vi "2D__Scaner+FM_v.9.6-ESP32.vi"() -> ()   [LabVIEW 2018]
uses:
  <vilib>/Analysis/Matrix/Datatypes/RealMatrix.ctl
  <vilib>/Platform/TimedLoop/XDataNode/timing_clust.ctl
  <vilib>/Platform/TimedLoop/XDataNode/nitl_modes.ctl
  <vilib>/Platform/TimedLoop/XDataNode/wakeup.ctl
  GlobalStop.vi
  <vilib>/Platform/TimedLoop/XDataNode/XDataNode.xnode
  <vilib>/Platform/TimedLoop/XDataNode/XDNodeRunTimeDep.lvlib
  <vilib>/Analysis/Matrix/NI_Matrix.lvlib
panel:
  out "Hour":i32 caption="Оставшееся время"
  out "Min":i32 caption="Оставшееся время"
  in  "Att":dbl(ring)=1.0 caption="Аттенюатор" items=["None"=1.0, "1%"=100.0, "3%"=34.0, "10%"=13.5, "30%"=4.6, "1+3%"=3400.0, "1+10%"=1350.0, "1+30%"=460.0, "3+10%"=459.0, "3+30%"=156.4, "10+30%"=62.1, "1+3+10%"=45900.0, "1+3+30%"=15640.0, "1+10+30%"=6210.0, "3+10+30%"=2111.4, "All"=211140.0]
  in  "Reboot ESP":bool
  out "Dir_x":bool
  out "Y_iter":i32
  in  "X_iter":i32
  in  "calc fi":bool=TRUE caption="Пересчет\nX в fi"
  out "pos_xy":cluster{"pos_x":dbl, "pos_y":dbl} caption="Позиция 2D, мм"
  in  "Mode initial 2D":enum32{"2D", "X"}(radio)=enum."X"
  out "pos_sample":dbl caption="Позиция FM с образцом"
  out "pos_no_sample":dbl caption="Позиция FM без образца"
  in  "Check pos":bool
  out "Sec":i32 caption="Оставшееся время"
  in  "Режим\nсканирования":enum32{"Ampl", "Phase"}(radio)
  out "st_joy":bool
  in  "Джостик":bool
  in  "Left":bool
  in  "Up":bool
  in  "Down":bool
  in  "Right":bool
  in  "Шаг, мкм":dbl=10000.0
  in  "Find pp":bool
  in  "Толщина образца":dbl min=0.0
  out "P_ref":dbl caption="Опорный сигнал \nс детектора"
  out "error sign.detect":errorcluster
  out "error esp-32":errorcluster
  out "COM-port":refnum<visa-resource-name>
  in  "COM-port ESP-32":refnum<visa-resource-name>="COM3"
  out "error out":errorcluster
  in  "error in (no error)":errorcluster
  in  "read signal?":bool
  in  "К позиции FM":i32=1000
  in  "Rotate FM":bool
  out "pos_z":dbl caption="Позиция FM"
  in  "Initial FM":bool
  out "График интенсивности":dbl[][](graph)
  in  "стоп":bool
  out "Завершено, %":dbl(slide) scale=0.0..100.0
  in  "Шаг по X":u32(knob)=1000 max=20000 scale=1.0..1000.0 scale format="%.0p"
  in  "начало Y, мм":dbl
  in  "начало X, мм":dbl
  in  "конец Y, мм":dbl=1.0
  in  "конец X, мм":dbl=1.0
  out "Результат сканирования":T1
  in  "Комментарий к файлу":string=" "
  in  "отмена":bool
  in  "сохр":bool
  in  "Имя файла с результатами":path=path "results.lvm" caption="Filename"
  in  "start scaning":bool
  in  "Шаг по Y":u32(knob)=1000 max=10000 scale=10.0..1000.0 scale format="%3.0p"
  out "Диалоговое окно":string
  in  "Initial 2D":bool
  in  "Частота излучения":dbl min=0.001
  # "Оставшееся время"
  # "м"
  # "с"
  # "ч"
  # "мм"
  # "Параметры сканирования"
  # "Начальная \nпозиция"
  # "ГГц"
  # "Область\nсканирования"
  # "мкм"
  # "Конечная\nпозиция"
  # "мм"
  # "мм"
  # "мм"
  # "мкм"
  # "мкм"
  # "мкм"
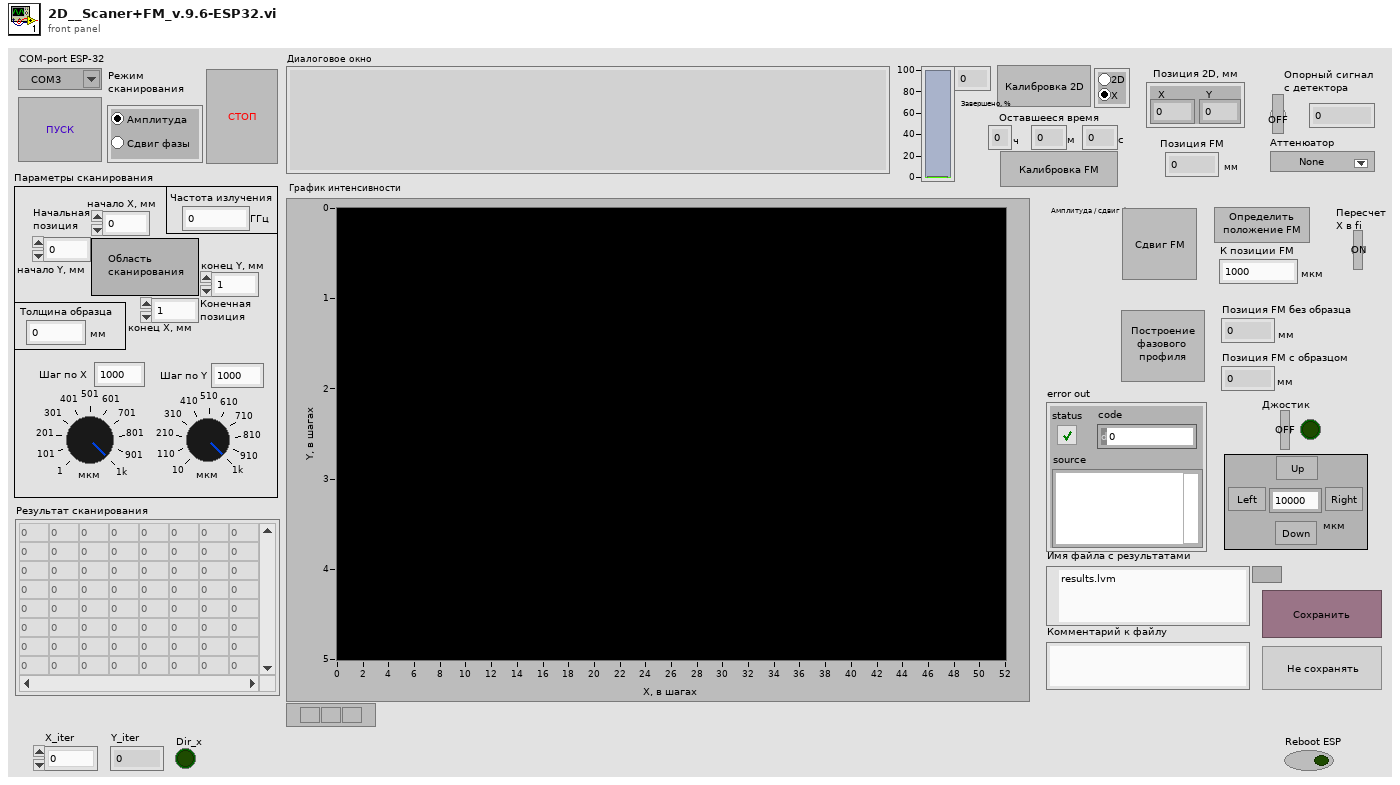
[diagram p1: front panel]
types:
  T1 = typedef "NI_Matrix.lvlib/RealMatrix.ctl" = dbl[][]
  T2 = typedef "XDNodeRunTimeDep.lvlib/timing_clust.ctl" = cluster{"Expected End [f-1]":u64, "Actual End [f-1]":u64, "Finished Late? [f-1]":bool, "Expected End [i-1]":u64, "Actual End [i-1]":u64, "Finished Late? [i-1]":bool, "Expected Start [i]":u64, "Actual Start [i]":u64, "Expected Start [f]":u64, "Actual Start [f]":u64, "Source Name":string, "Structure Name":string, "Period":i64, "Deadline":i64, "Offset":i64, "Start":i64, "Priority":i32, "Timeout":i32, "Mode":T3, "Wakeup Reason":T4, "Error":errorcluster, "Source Type":string, "Secondary Source Type":string, "Global End Time":u64, "Global Start Time":u64, "Frame Duration":u64, "Iteration Duration":u64, "Assigned CPU":i32, "I/O Scan Engine Mode":u32}
  T3 = typedef "XDNodeRunTimeDep.lvlib/nitl_modes.ctl" = enum32{"No Change", "Process missed periods, maintain original phase", "Discard missed periods, maintain original phase", "Process missed periods, ignore original phase", "Discard missed periods, ignore original phase"}
  T4 = typedef "XDNodeRunTimeDep.lvlib/wakeup.ctl" = enum32{"Normal", "Aborted", "Asynchronous wakeup", "Timing source error", "Timed loop error", "Timeout"}
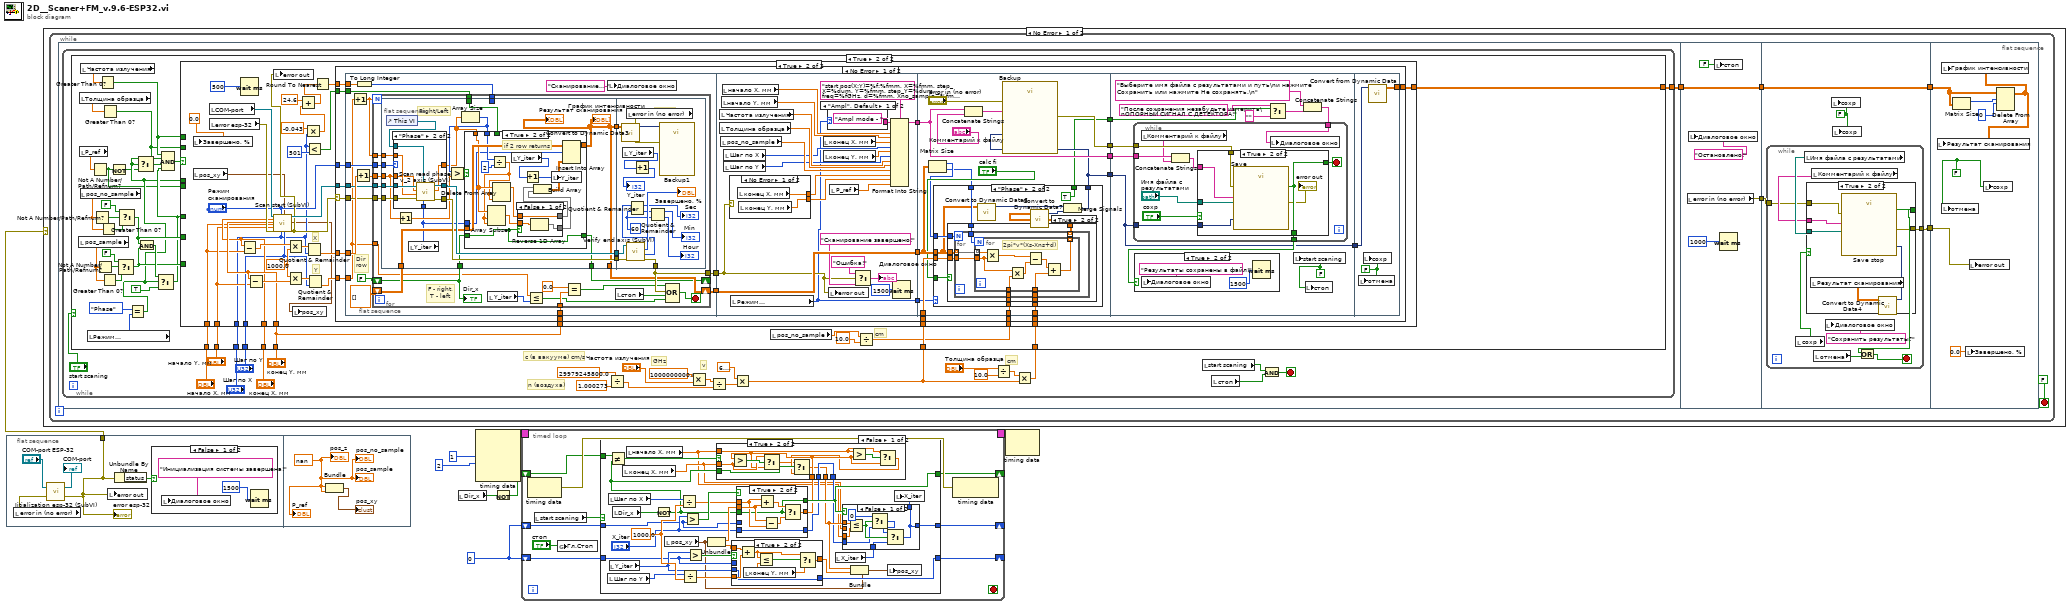
[diagram p0: block diagram]
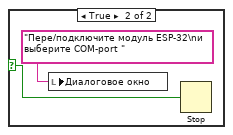
[diagram p2: hidden frame]
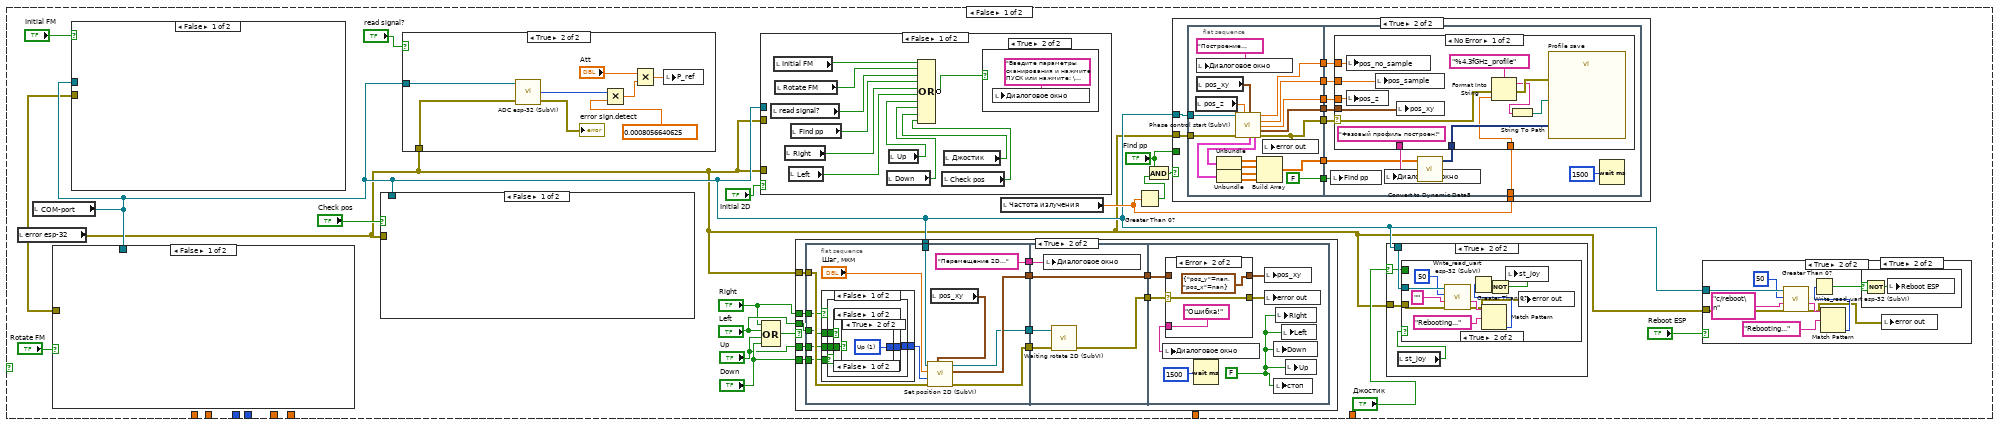
[diagram p3: hidden frame]
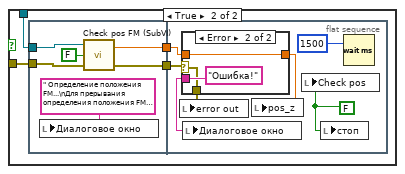
[diagram p6: hidden frame]
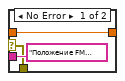
[diagram p7: hidden frame]
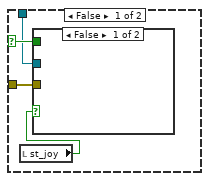
[diagram p8: hidden frame]
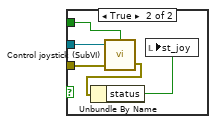
[diagram p9: hidden frame]
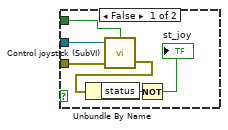
[diagram p10: hidden frame]
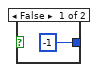
[diagram p12: hidden frame]
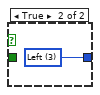
[diagram p13: hidden frame]
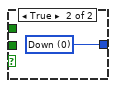
[diagram p14: hidden frame]
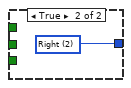
[diagram p15: hidden frame]
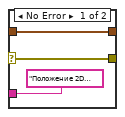
[diagram p16: hidden frame]
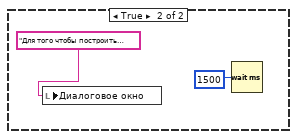
[diagram p18: hidden frame]
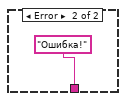
[diagram p19: hidden frame]
diagram:
  w3 = 0 ("Y_iter")
  n1 = flat-sequence {
    tunnel: [w9] -> w6
    frame #0 {
      n2 = local read "error in (no error)"() -> (w11:errorcluster)
      n3 = call "Iitialization esp-32 (SubVI).vi"("error in (no error)"=w11, "COM-port"="COM-port ESP-32") -> ("error out"=w9:errorcluster, "COM-port out"=→"COM-port":refnum<visa-resource-name>)
      "error esp-32" <- w9
      n4 = local write "error out"(w9) -> ()
      n5 = Unbundle By Name(w9) -> ("status"=w10:bool)
      n6 = case shown="False" w10 {
        selector: w10 -> [_ w16]
        frame False {
          n7 = local write "Диалоговое окно"("Инициализация системы завершена!" ("Диалоговое окно")) -> ()
          n8 = Wait (ms)(milliseconds to wait=u32 1500) -> ()  [unwired: 1 out]
        }
        frame True {
          n9 = local write "Диалоговое окно"("Пере/подключите модуль ESP-32\nи выберите COM-port " ("t")) -> ()
          n10 = Stop(stop? (T)=w16) -> ()
        }
      }
    }
    frame #1 {
      w19 = nan
      n11 = Bundle(w19, w19) -> (→"pos_xy":cluster{dbl, dbl})  [unwired: 1 in]
      "pos_z" <- w19
      "P_ref" <- w19
      "pos_no_sample" <- w19
      "pos_sample" <- w19
    }
  }
  n12 = case shown="No Error" w6 {
    frame No Error {
      n13 = while {
        stop <- FALSE stop-if-true
        n14 = flat-sequence {
          tunnel: [w26] -> w22
          tunnel: w22 -> [w723]
          tunnel: [w723] -> w21
          tunnel: [w719] -> w20
          tunnel: [w727] -> w25
          tunnel: w21 -> [w727]
          tunnel: w20 -> [w725]
          tunnel: [w724] -> w23
          tunnel: w25 -> [w750]
          tunnel: w23 -> [w747]
          frame #0 {
            n15 = while {
              tunnel: [w49] -> w26
              stop <- w38 stop-if-true
              # "cm"
              # "v"
              # "GHz"
              # "n (воздуха)"
              # "c (в вакууме) cm/s"
              n16 = Divide(x=29979245800.0, y=1.000273) -> (x/y=w43:dbl)
              n17 = Multiply(x=1000000000.0, y="Частота излучения") -> (x*y=w34:dbl)
              n18 = Divide(x=w34, y=w43) -> (x/y=w31:dbl)
              n19 = Multiply(x=6.283185307179586, y=w31) -> (x*y=w32:dbl)
              n20 = Divide(x="Толщина образца", y=10.0) -> (x/y=w29:dbl)
              n21 = Multiply(x=w29, y=w32) -> (x*y=w42:dbl)
              n22 = case shown="True" "start scaning" {
                tunnel: "конец Y, мм" -> [_ w341]
                tunnel: "конец X, мм" -> [_ w346]
                tunnel: "начало Y, мм" -> [_ w343]
                tunnel: "начало X, мм" -> [_ w342]
                tunnel: [_ w371] -> w49
                tunnel: w32 -> [_ w370]
                tunnel: w42 -> [_ w369]
                tunnel: "Шаг по X" -> [_ w344]
                tunnel: "Шаг по Y" -> [_ w345]
                frame False {
                  n23 = local read "error esp-32"() -> (w51:errorcluster)
                  n24 = local read "COM-port"() -> (w52:refnum<visa-resource-name>)
                  n25 = case shown="False" "Rotate FM" {
                    tunnel: w52 -> [_ w256]
                    tunnel: w51 -> [_ w252]
                    frame False {
                    }
                    frame True {
                      n26 = flat-sequence {
                        tunnel: w256 -> [w264]
                        tunnel: w252 -> [w258]
                        tunnel: [w262] -> w255
                        tunnel: [w261] -> w254
                        tunnel: [FALSE ("Rotate FM")] -> w253
                        tunnel: w255 -> [w267]
                        tunnel: w254 -> [w266]
                        tunnel: w253 -> [w265]
                        frame #0 {
                          n27 = local write "Диалоговое окно"("Перемещение FM...\nДля прерывания перемещения FM нажмите на Джостик!" ("Диалоговое окно")) -> ()
                          n28 = local read "pos_z"() -> (w259:dbl)
                          n29 = call "Set position FM (SubVI).vi"("VISA Refnum in"=w264, "Позиция, мкм"="К позиции FM", "error in"=w258, "pos_z"=w259) -> ("set_pos_z"=w262:dbl, "error out"=w261:errorcluster)  [unwired: 2 in]
                        }
                        frame #1 {
                          n30 = local write "Rotate FM"(w265) -> ()
                          n31 = case shown="No Error" w266 {
                            selector: w266 -> [w272 w275]
                            tunnel: ["Положение FM достигнуто!" ("Диалоговое окно") "Ошибка!" ("Диалоговое окно")] -> w270
                            tunnel: w267 -> [w273 _]
                            tunnel: [w273 nan ("set_pos_x")] -> w268
                            tunnel: [w272 w275] -> w269
                            frame No Error {
                            }
                            frame Error {
                            }
                          }
                          n32 = local write "Диалоговое окно"(w270) -> ()
                          n33 = local write "error out"(w269) -> ()
                          n34 = local write "стоп"(w265) -> ()
                          n35 = local write "pos_z"(w268) -> ()
                          n36 = Wait (ms)(milliseconds to wait=u32 1500) -> ()  [unwired: 1 out]
                        }
                      }
                    }
                  }
                  n37 = case shown="False" "Initial FM" {
                    tunnel: w51 -> [_ w282]
                    tunnel: w52 -> [_ w281]
                    frame False {
                    }
                    frame True {
                      n38 = flat-sequence {
                        tunnel: w282 -> [w287]
                        tunnel: w281 -> [w286]
                        tunnel: [w285] -> w280
                        tunnel: [FALSE ("Initial FM")] -> w279
                        tunnel: [u32 1500 ("milliseconds to wait")] -> w278
                        tunnel: w280 -> [w292]
                        tunnel: w279 -> [w289]
                        tunnel: w278 -> [w291]
                        frame #0 {
                          n39 = local write "Диалоговое окно"("Калибровка FM...\nДля прерывания калибровки FM нажмите на Джостик!" ("Диалоговое окно")) -> ()
                          n40 = call "Initial Z (SubVI).vi"("error in (no error)"=w287, "VISA Refnum in"=w286) -> ("error out"=w285:errorcluster)  [unwired: 1 in]
                        }
                        frame #1 {
                          n41 = Wait (ms)(milliseconds to wait=w291) -> ()  [unwired: 1 out]
                          n42 = case shown="No Error" w292 {
                            selector: w292 -> [w297 w300]
                            tunnel: [w297 w300] -> w294
                            tunnel: ["Калибровка завершена!" ("Диалоговое окно") "Ошибка!" ("Диалоговое окно")] -> w290
                            tunnel: [0.0 nan] -> w293
                            frame No Error {
                            }
                            frame Error {
                            }
                          }
                          n43 = local write "Initial FM"(w289) -> ()
                          n44 = local write "Диалоговое окно"(w290) -> ()
                          n45 = local write "pos_z"(w293) -> ()
                          n46 = local write "стоп"(w289) -> ()
                          n47 = local write "error out"(w294) -> ()
                        }
                      }
                    }
                  }
                  n48 = case shown="False" "Check pos" {
                    tunnel: w52 -> [_ w83]
                    tunnel: w51 -> [_ w82]
                    frame False {
                    }
                    frame True {
                      n49 = flat-sequence {
                        tunnel: w83 -> [w89]
                        tunnel: w82 -> [w88]
                        tunnel: [w87] -> w81
                        tunnel: [w86] -> w80
                        tunnel: w81 -> [w96]
                        tunnel: w80 -> [w95]
                        frame #0 {
                          n50 = local write "Диалоговое окно"(" Определение положения FM...\nДля прерывания определения положения FM нажмите на Джостик!" ("Диалоговое окно")) -> ()
                          n51 = call "Check pos FM (SubVI).vi"("error in"=w88, "verify?"=FALSE, "VISA Refnum in"=w89) -> ("error out"=w87:errorcluster, "position"=w86:dbl)
                        }
                        frame #1 {
                          w91 = FALSE
                          n52 = case shown="Error" w96 {
                            selector: w96 -> [w98 w101]
                            tunnel: ["Положение FM определено!" ("Диалоговое окно") "Ошибка!" ("Диалоговое окно")] -> w93
                            tunnel: [w97 w100] -> w94
                            tunnel: [w98 w101] -> w90
                            tunnel: w95 -> [w97 w100]
                            frame No Error {
                            }
                            frame Error {
                            }
                          }
                          n53 = local write "error out"(w90) -> ()
                          n54 = local write "Диалоговое окно"(w93) -> ()
                          n55 = local write "pos_z"(w94) -> ()
                          n56 = local write "Check pos"(w91) -> ()
                          n57 = local write "стоп"(w91) -> ()
                          n58 = Wait (ms)(milliseconds to wait=u32 1500) -> ()  [unwired: 1 out]
                        }
                      }
                    }
                  }
                  n59 = case shown="True" "read signal?" {
                    tunnel: w52 -> [_ w248]
                    tunnel: w51 -> [_ w247]
                    frame False {
                    }
                    frame True {
                      n60 = call "ADC esp-32 (SubVI).vi"("error in (no error)"=w247, "VISA Refnum in"=w248) -> ("error out"=→"error sign.detect":errorcluster, "value adc"=w249:i16)  [unwired: 1 in, 1 out]
                      n61 = Multiply(x=w249, y=0.0008056640625) -> (x*y=w245:dbl)
                      n62 = Multiply(x="Att", y=w245) -> (x*y=w244:dbl)
                      n63 = local write "P_ref"(w244) -> ()
                    }
                  }
                  n64 = case shown="False" "Initial 2D" {
                    tunnel: w52 -> [_ w317]
                    tunnel: w51 -> [_ _]
                    tunnel: w51 -> [_ w316]
                    frame False {
                      n65 = local read "read signal?"() -> (w308:bool)
                      n66 = local read "Initial FM"() -> (w310:bool)
                      n67 = local read "Rotate FM"() -> (w309:bool)
                      n68 = local read "Right"() -> (w306:bool)
                      n69 = local read "Left"() -> (w305:bool)
                      n70 = local read "Find pp"() -> (w307:bool)
                      n71 = local read "Down"() -> (w303:bool)
                      n72 = local read "Up"() -> (w304:bool)
                      n73 = local read "Check pos"() -> (w301:bool)
                      n74 = local read "Джостик"() -> (w302:bool)
                      n75 = Compound Arithmetic op=OR(w310, w309, w308, w307, w306, w305, w304, w303, w302, w301) -> (invert w311:bool)
                      n76 = case shown="True" w311 {
                        frame False {
                        }
                        frame True {
                          n77 = local write "Диалоговое окно"("Введите параметры сканирования и нажмите ПУСК или нажмите: \nКалибровка 2D (крайнее левое верхнее положение), Калибровка FM \n(крайнее правое положение), Сдвиг FM (на требуемую позицию),\nНайти положение FM c мин. сигналом, ON/OFF - Сигнал с детектора " ("Диалоговое окно")) -> ()
                        }
                      }
                    }
                    frame True {
                      n78 = flat-sequence {
                        tunnel: w316 -> [w322]
                        tunnel: w317 -> [w321]
                        tunnel: [w319] -> w315
                        tunnel: w315 -> [w328]
                        tunnel: [w327] -> w314
                        tunnel: [w323] -> w313
                        frame #0 {
                          n79 = local write "Диалоговое окно"("Калибровка 2D...\nДля прерывания калибровки 2D нажмите на Джостик!" ("Диалоговое окно")) -> ()
                          n80 = call "Initial XY (SubVI).vi"("Mode initial 2D"="Mode initial 2D", "error in"=w322, "VISA Refnum in"=w321) -> ("error out"=w319:errorcluster)
                        }
                        frame #1 {
                          w326 = FALSE ("Гл.Стоп")
                          n81 = case shown="No Error" w328 {
                            selector: w328 -> [w331 w334]
                            tunnel: [w331 w334] -> w327
                            tunnel: ["Калибровка завершена!" ("Диалоговое окно") "Ошибка!" ("Диалоговое окно")] -> w324
                            tunnel: [cluster{"pos_y":dbl, "pos_x":dbl} {"pos_y"=0.0, "pos_x"=0.0} ("pos_xy") cluster{"pos_y":dbl, "pos_x":dbl} {"pos_y"=nan, "pos_x"=nan} ("pos_xy")] -> w323
                            frame No Error {
                            }
                            frame Error {
                            }
                          }
                          n82 = local write "Initial 2D"(w326) -> ()
                          n83 = local write "Диалоговое окно"(w324) -> ()
                          n84 = Wait (ms)(milliseconds to wait=u32 1500) -> ()  [unwired: 1 out]
                          n85 = local write "стоп"(w326) -> ()
                        }
                      }
                      n86 = local write "error out"(w314) -> ()
                      n87 = local write "pos_xy"(w313) -> ()
                    }
                  }
                  n88 = Compound Arithmetic op=OR("Right", "Left", "Up", "Down") -> (w64:bool)
                  n89 = case shown="True" w64 {
                    tunnel: w52 -> [_ w143]
                    tunnel: w51 -> [_ w142]
                    tunnel: "Right" -> [_ w135]
                    tunnel: "Down" -> [_ w134]
                    tunnel: "Left" -> [_ w133]
                    tunnel: "Up" -> [_ w132]
                    frame False {
                    }
                    frame True {
                      n90 = flat-sequence {
                        tunnel: w143 -> [w146]
                        tunnel: w142 -> [w155]
                        tunnel: [w154] -> w140
                        tunnel: ["Перемещение 2D..." ("Диалоговое окно")] -> w138
                        tunnel: [w152] -> w137
                        tunnel: [w151] -> w136
                        tunnel: w135 -> [w150]
                        tunnel: w134 -> [w149]
                        tunnel: w133 -> [w148]
                        tunnel: w132 -> [w147]
                        tunnel: [w172] -> w141
                        tunnel: w140 -> [w175]
                        tunnel: [w175] -> w139
                        tunnel: w138 -> [w174]
                        tunnel: w137 -> [w173]
                        tunnel: w136 -> [w171]
                        tunnel: w141 -> [w180]
                        tunnel: w139 -> [w179]
                        frame #0 {
                          n91 = case shown="False" w150 {
                            tunnel: w149 -> [w160 _]
                            tunnel: [w159 w170] -> w145
                            tunnel: w148 -> [w158 _]
                            tunnel: w147 -> [w157 _]
                            frame False {
                              n92 = case shown="False" w160 {
                                tunnel: [w162 w169] -> w159
                                tunnel: w158 -> [w163 _]
                                tunnel: w157 -> [w161 _]
                                frame False {
                                n93 = case shown="False" w163 {
                                tunnel: [w164 w168] -> w162
                                tunnel: w161 -> [w165 _]
                                frame False {
                                n94 = case shown="True" w165 {
                                tunnel: [-1 w167] -> w164
                                frame False {
                                }
                                frame True {
                                w167 = u16 1 items=["Down", "Up", "Right", "Left"] ("Direct")
                                }
                                }
                                }
                                frame True {
                                w168 = u16 3 items=["Down", "Up", "Right", "Left"] ("Direct")
                                }
                                }
                                }
                                frame True {
                                w169 = u16 0 items=["Down", "Up", "Right", "Left"] ("Direct")
                                }
                              }
                            }
                            frame True {
                              w170 = u16 2 items=["Down", "Up", "Right", "Left"] ("Direct")
                            }
                          }
                          n95 = local read "pos_xy"() -> (w144:cluster{"pos_x":dbl, "pos_y":dbl})
                          n96 = call "Set position 2D (SubVI).vi"("last_pos_xy"=w144, "error in"=w155, "Direct"=w145, "Шаг"="Шаг, мкм", "VISA Refnum in"=w146) -> ("error out"=w152:errorcluster, "set_pos_xy"=w154:cluster{"pos_x":dbl, "pos_y":dbl}, "VISA Refnum out"=w151:refnum<visa-resource-name>)  [unwired: 2 in]
                        }
                        frame #1 {
                          n97 = local write "Диалоговое окно"(w174) -> ()
                          n98 = call "Waiting rotate 2D (SubVI).vi"("error in (no error)"=w173, "VISA Refnum in"=w171) -> ("error out"=w172:errorcluster)  [unwired: 3 in]
                        }
                        frame #2 {
                          w177 = FALSE ("Go 2D")
                          n99 = case shown="Error" w180 {
                            selector: w180 -> [w184 w187]
                            tunnel: ["Положение 2D достигнуто!" ("Диалоговое окно") "Ошибка!" ("Диалоговое окно")] -> w181
                            tunnel: w179 -> [w183 _]
                            tunnel: [w184 w187] -> w178
                            tunnel: [w183 cluster{"pos_y":dbl, "pos_x":dbl} {"pos_y"=nan, "pos_x"=nan} ("set_pos_xy")] -> w176
                            frame No Error {
                            }
                            frame Error {
                            }
                          }
                          n100 = local write "Диалоговое окно"(w181) -> ()
                          n101 = Wait (ms)(milliseconds to wait=u32 1500) -> ()  [unwired: 1 out]
                          n102 = local write "pos_xy"(w176) -> ()
                          n103 = local write "error out"(w178) -> ()
                          n104 = local write "Down"(w177) -> ()
                          n105 = local write "стоп"(w177) -> ()
                          n106 = local write "Right"(w177) -> ()
                          n107 = local write "Left"(w177) -> ()
                          n108 = local write "Up"(w177) -> ()
                        }
                      }
                    }
                  }
                  n109 = local read "Частота излучения"() -> (w55:dbl)
                  n110 = Greater Than 0?(x=w55) -> (x > 0?=w56:bool)
                  n111 = And(x="Find pp", y=w56) -> (x .and. y?=w57:bool)
                  n112 = case shown="True" w57 {
                    tunnel: w52 -> [_ w199]
                    tunnel: w51 -> [_ w200]
                    tunnel: w55 -> [_ w192]
                    tunnel: "Find pp" -> [w189 _]
                    frame False {
                      n113 = case shown="False" w189 {
                        frame False {
                        }
                        frame True {
                          n114 = local write "Диалоговое окно"("Для того чтобы построить фазовый профиль введите Частоту излучения" ("Диалоговое окно")) -> ()
                          n115 = Wait (ms)(milliseconds to wait=u32 1500) -> ()  [unwired: 1 out]
                        }
                      }
                    }
                    frame True {
                      n116 = flat-sequence {
                        tunnel: w200 -> [w219]
                        tunnel: [w214] -> w201
                        tunnel: w199 -> [w217]
                        tunnel: [w213] -> w198
                        tunnel: [w212] -> w197
                        tunnel: [w211] -> w196
                        tunnel: [w210] -> w195
                        tunnel: [FALSE ("Find phase prifile")] -> w194
                        tunnel: [w202] -> w193
                        tunnel: w201 -> [w228]
                        tunnel: w198 -> [w227]
                        tunnel: w197 -> [w226]
                        tunnel: w196 -> [w225]
                        tunnel: w195 -> [w224]
                        tunnel: w194 -> [w223]
                        tunnel: w193 -> [w221]
                        tunnel: w192 -> [w220]
                        frame #0 {
                          n117 = local read "pos_z"() -> (w215:dbl)
                          n118 = local write "Диалоговое окно"("Построение профиля..." ("Диалоговое окно")) -> ()
                          n119 = local read "pos_xy"() -> (w216:cluster{"pos_x":dbl, "pos_y":dbl})
                          n120 = call "Phase control start (SubVI).vi"("VISA Refnum in"=w217, "pos_z_in"=w215, "pos_xy_in"=w216, "error in"=w219) -> ("pos_no_sample"=w210:dbl, "pos_sample"=w211:dbl, "pos_z_out"=w212:dbl, "pos_xy_out"=w213:cluster{"pos_y":dbl, "pos_x":dbl}, "Profile_ns out"=w208:cluster{dbl[], dbl[]}, "Profile_s out"=w207:cluster{dbl[], dbl[]}, "error out"=w214:errorcluster)  [unwired: 5 in]
                          n121 = Unbundle(w207) -> (w206:dbl[], w205:dbl[])
                          n122 = Unbundle(w208) -> (w204:dbl[], w203:dbl[])
                          n123 = Build Array(w206, w205, w204, w203) -> (w202:dbl[][])
                          n124 = local write "error out"(w214) -> ()
                        }
                        frame #1 {
                          n125 = local write "Find pp"(w223) -> ()
                          n126 = call "Convert to Dynamic Data5"("2D Array"=w221) -> ("Dynamic Data Type"=w222:dynamicdata)  [unwired: 3 in]
                          n127 = case shown="No Error" w228 {
                            selector: w228 -> [w234 _]
                            tunnel: ["Фазовый профиль построен!" ("Диалоговое окно") "Ошибка!" ("Диалоговое окно")] -> w229
                            tunnel: w227 -> [w241 _]
                            tunnel: w226 -> [w240 _]
                            tunnel: w225 -> [w239 _]
                            tunnel: w224 -> [w238 _]
                            tunnel: w222 -> [w237 _]
                            tunnel: w220 -> [w235 _]
                            frame No Error {
                              n128 = local write "pos_no_sample"(w238) -> ()
                              n129 = local write "pos_z"(w240) -> ()
                              n130 = local write "pos_sample"(w239) -> ()
                              n131 = local write "pos_xy"(w241) -> ()
                              n132 = Format Into String(format string="%4.3fGHz_profile", error in=w234, w235) -> (resulting string=w232:string, error out=w233:errorcluster)  [unwired: 1 in]
                              n133 = String To Path(string=w232) -> (path=w231:path)
                              n134 = call "Profile save"("Signals"=w237, "error in (no error)"=w233, "Filename"=w231) -> ()  [unwired: 14 in, 3 out]
                            }
                            frame Error {
                            }
                          }
                          n135 = local write "Диалоговое окно"(w229) -> ()
                          n136 = Wait (ms)(milliseconds to wait=u32 1500) -> ()  [unwired: 1 out]
                        }
                      }
                    }
                  }
                  n137 = case shown="True" "Джостик" {
                    selector: "Джостик" -> [w106 w113]
                    tunnel: w52 -> [w105 w115]
                    tunnel: w51 -> [w104 w114]
                    frame False {
                      n138 = local read "st_joy"() -> (w103:bool)
                      n139 = case shown="False" w103 {
                        tunnel: w106 -> [_ w110]
                        tunnel: w105 -> [_ w111]
                        tunnel: w104 -> [_ w109]
                        frame False {
                        }
                        frame True {
                          n140 = call "Control joystick (SubVI).vi"("Start/stop"=w110, "error in (no error)"=w109, "VISA Refnum in"=w111) -> ("error out"=w108:errorcluster)  [unwired: 1 in, 1 out]
                          n141 = Unbundle By Name(w108) -> ("status"=w107:bool)
                          n142 = local write "st_joy"(w107) -> ()
                        }
                      }
                    }
                    frame True {
                      n143 = local read "st_joy"() -> (w112:bool)
                      n144 = case shown="True" w112 {
                        tunnel: w115 -> [w121 w131]
                        tunnel: w114 -> [w120 w130]
                        tunnel: w113 -> [w116 _]
                        frame False {
                          n145 = call "Control joystick (SubVI).vi"("Start/stop"=w116, "error in (no error)"=w120, "VISA Refnum in"=w121) -> ("error out"=w119:errorcluster)  [unwired: 1 in, 1 out]
                          n146 = Unbundle By Name(w119) -> ("status"=w117:bool)
                          n147 = Not(x=w117) -> (.not. x?=→"st_joy":bool)
                        }
                        frame True {
                          n148 = call "Write_read_uart esp-32 (SubVI).vi"("error in (no error)"=w130, "write buffer"="", "milliseconds to wait"=u32 50, "VISA Refnum in"=w131) -> ("error out 4"=w122:errorcluster, "read buffer"=w127:string)  [unwired: 2 out]
                          n149 = Match Pattern(string=w127, regular expression="Rebooting...") -> (offset past match=w125:i32)  [unwired: 1 in, 3 out]
                          n150 = Greater Than 0?(x=w125) -> (x > 0?=w124:bool)
                          n151 = Not(x=w124) -> (.not. x?=w123:bool)
                          n152 = local write "st_joy"(w123) -> ()
                          n153 = local write "error out"(w122) -> ()
                        }
                      }
                    }
                  }
                  n154 = case shown="True" "Reboot ESP" {
                    tunnel: w52 -> [_ w77]
                    tunnel: w51 -> [_ w70]
                    frame False {
                    }
                    frame True {
                      n155 = call "Write_read_uart esp-32 (SubVI).vi"("error in (no error)"=w70, "write buffer"="c/reboot\n", "milliseconds to wait"=u32 50, "VISA Refnum in"=w77) -> ("error out 4"=w71:errorcluster, "read buffer"=w74:string)  [unwired: 2 out]
                      n156 = Match Pattern(string=w74, regular expression="Rebooting...") -> (offset past match=w72:i32)  [unwired: 1 in, 3 out]
                      n157 = Greater Than 0?(x=w72) -> (x > 0?=w69:bool)
                      n158 = case shown="True" w69 {
                        selector: w69 -> [_ w78]
                        frame False {
                        }
                        frame True {
                          n159 = Not(x=w78) -> (.not. x?=w79:bool)
                          n160 = local write "Reboot ESP"(w79) -> ()
                        }
                      }
                      n161 = local write "error out"(w71) -> ()
                    }
                  }
                }
                frame True {
                  # "cm"
                  n162 = local read "pos_sample"() -> (w361:dbl)
                  n163 = local read "Толщина образца"() -> (w347:dbl)
                  n164 = local read "P_ref"() -> (w340:dbl)
                  n165 = local read "pos_no_sample"() -> (w363:dbl)
                  n166 = local read "Частота излучения"() -> (w368:dbl)
                  n167 = local read "Режим\nсканирования"() -> (w356:enum32{"Ampl", "Phase"})
                  n168 = Not A Number/Path/Refnum?(number/path/refnum=w340) -> (NaN/Path/Refnum?=w335:bool)
                  n169 = Not A Number/Path/Refnum?(number/path/refnum=w363) -> (NaN/Path/Refnum?=w366:bool)
                  n170 = Not A Number/Path/Refnum?(number/path/refnum=w361) -> (NaN/Path/Refnum?=w367:bool)
                  n171 = Greater Than 0?(x=w368) -> (x > 0?=w358:bool)
                  n172 = Greater Than 0?(x=w363) -> (x > 0?=w362:bool)
                  n173 = Greater Than 0?(x=w361) -> (x > 0?=w360:bool)
                  n174 = Greater Than 0?(x=w347) -> (x > 0?=w357:bool)
                  n175 = Not(x=w335) -> (.not. x?=w336:bool)
                  n176 = Select(t=FALSE, s=w367, f=w360) -> (s? t:f=w348:bool)
                  n177 = Select(t=FALSE, s=w366, f=w362) -> (s? t:f=w349:bool)
                  n178 = Equal?(x=enum32{"Ampl", "Phase"}."Phase", y=w356) -> (x = y?=w337:bool)
                  n179 = Select(t=w337, s=w337, f=w336) -> (s? t:f=w338:bool)
                  n180 = And(x=w349, y=w348) -> (x .and. y?=w353:bool)
                  n181 = Select(t=w353, s=w337, f=TRUE) -> (s? t:f=w339:bool)
                  n182 = Compound Arithmetic op=AND(w358, w357, w338, w339) -> (w359:bool)
                  n183 = local read "pos_no_sample"() -> (w351:dbl)
                  n184 = Divide(x=w351, y=10.0) -> (x/y=w350:dbl)
                  n185 = case shown="True" w359 {
                    tunnel: [dbl[][] [] ("Intensity Graph") w445] -> w371
                    tunnel: w370 -> [_ w444]
                    tunnel: w369 -> [_ w443]
                    tunnel: w358 -> [w410 _]
                    tunnel: w357 -> [w408 _]
                    tunnel: w339 -> [w401 _]
                    tunnel: w349 -> [w400 _]
                    tunnel: w348 -> [w399 _]
                    tunnel: w350 -> [_ w442]
                    tunnel: w341 -> [_ w432]
                    tunnel: w346 -> [_ w431]
                    tunnel: w345 -> [_ w430]
                    tunnel: w344 -> [_ w419]
                    tunnel: w343 -> [_ w429]
                    tunnel: w342 -> [_ w428]
                    tunnel: w341 -> [_ w412]
                    tunnel: w337 -> [w379 _]
                    tunnel: w335 -> [w378 _]
                    frame False {
                      w375 = "" ("f")
                      w402 = "" ("f")
                      n186 = Not(x=w410) -> (.not. x?=w381:bool)
                      n187 = Not(x=w408) -> (.not. x?=w382:bool)
                      n188 = Select(t=FALSE, s=w379, f=w378) -> (s? t:f=w377:bool)
                      n189 = Select(t=" Частота излучения ", s=w381, f=w402) -> (s? t:f=w406:string)
                      n190 = Or(x=w381, y=w382) -> (x .or. y?=w411:bool)
                      n191 = Not(x=w399) -> (.not. x?=w383:bool)
                      n192 = Select(t="\nНеобходимо зафиксировать величину опорного сигнала с детектора!", s=w377, f=w375) -> (s? t:f=w373:string)
                      n193 = Not(x=w400) -> (.not. x?=w384:bool)
                      n194 = Select(t=" Толщина образца ", s=w382, f=w402) -> (s? t:f=w405:string)
                      n195 = Select(t=" Без образца ", s=w384, f=w375) -> (s? t:f=w395:string)
                      n196 = Select(t=" С образцом ", s=w383, f=w375) -> (s? t:f=w394:string)
                      n197 = Concatenate Strings("Проверьте правильность ввода праметров: ", w406, w405) -> (w403:string)
                      n198 = Concatenate Strings("\nНеобходимо определить положение FM: ", w395, w394) -> (w393:string)
                      n199 = Select(t=w375, s=w401, f=w393) -> (s? t:f=w374:string)
                      n200 = Select(t=w403, s=w411, f=w402) -> (s? t:f=w392:string)
                      n201 = Concatenate Strings(w392, w373, w374) -> (w380:string)
                      n202 = local write "Диалоговое окно"(w380) -> ()
                      n203 = local read "error in (no error)"() -> (w390:errorcluster)
                      n204 = Bundle(cluster=w390, "status"=TRUE, "code"=-1, "source"=w380) -> (w387:errorcluster)
                      n205 = local write "error out"(w387) -> ()
                      n206 = Wait (ms)(milliseconds to wait=u32 10000) -> ()  [unwired: 1 out]
                      n207 = local write "start scaning"(FALSE ("start scaning")) -> ()
                    }
                    frame True {
                      w437 = 1000.0 ("y")
                      # "X"
                      # "Y"
                      n208 = local write "Завершено, %"(0.0 ("Завершено, %")) -> ()
                      n209 = local read "pos_xy"() -> (w414:cluster{"pos_x":dbl, "pos_y":dbl})
                      n210 = local read "COM-port"() -> (w435:refnum<visa-resource-name>)
                      n211 = local read "error esp-32"() -> (w434:errorcluster)
                      n212 = Wait (ms)(milliseconds to wait=u32 500) -> ()  [unwired: 1 out]
                      n213 = Subtract(x=w431, y=w428) -> (x-y=w440:dbl)
                      n214 = Subtract(x=w432, y=w429) -> (x-y=w441:dbl)
                      n215 = call "Scan start (SubVI).vi"("VISA Refnum in"=w435, "end_x"=w431, "end_y"=w432, "sp_x"=w428, "sp_y"=w429, "error in"=w434, "Режим\nсканирования"="Режим\nсканирования", "step_x"=w419, "pos_xy"=w414, "step_y"=w430) -> ("VISA resource name out"=w425:refnum<visa-resource-name>, "set_pos_xy"=w413:cluster{"pos_x":dbl, "pos_y":dbl}, "error out"=w424:errorcluster)  [unwired: 7 in]
                      n216 = local write "error out"(w424) -> ()
                      n217 = Multiply(x=w440, y=w437) -> (x*y=w438:dbl)
                      n218 = Multiply(x=w437, y=w441) -> (x*y=w439:dbl)
                      n219 = local write "pos_xy"(w413) -> ()
                      n220 = Multiply(x=-0.043 ("y"), y=w419) -> (x*y=w417:dbl)
                      n221 = Add(x=24.6, y=w417) -> (x+y=w416:dbl)
                      n222 = Less?(x=w419, y=u32 501) -> (x < y?=w421:bool)
                      n223 = Quotient & Remainder(x=w438, y=w419) -> (floor(x/y)=w426:dbl)  [unwired: 1 out]
                      n224 = Quotient & Remainder(x=w439, y=w430) -> (floor(x/y)=w427:dbl)  [unwired: 1 out]
                      n225 = Round To Nearest(number=w416) -> (nearest integer value=w415:dbl)
                      n226 = case shown="No Error" w424 {
                        selector: w424 -> [w454 _]
                        tunnel: [w448 dbl[][] [] ("Intensity Graph")] -> w445
                        tunnel: w444 -> [w461 _]
                        tunnel: w443 -> [w460 _]
                        tunnel: w442 -> [w459 _]
                        tunnel: w427 -> [w458 _]
                        tunnel: w426 -> [w457 _]
                        tunnel: w425 -> [w456 _]
                        tunnel: "Режим\nсканирования" -> [w455 _]
                        tunnel: w421 -> [w453 _]
                        tunnel: w415 -> [w452 _]
                        tunnel: w412 -> [w451 _]
                        frame No Error {
                          n227 = flat-sequence {
                            tunnel: [w482] -> w467
                            tunnel: [w478] -> w466
                            tunnel: w458 -> [w468]
                            tunnel: w457 -> [w476]
                            tunnel: w454 -> [w475]
                            tunnel: w456 -> [w474]
                            tunnel: w455 -> [w473]
                            tunnel: w453 -> [w472]
                            tunnel: w452 -> [w471]
                            tunnel: w451 -> [w469]
                            tunnel: w467 -> [w621]
                            tunnel: [w621] -> w465
                            tunnel: [w620] -> w464
                            tunnel: w466 -> [w605]
                            tunnel: [w602] -> w463
                            tunnel: w465 -> [w644]
                            tunnel: w464 -> [w634]
                            tunnel: w461 -> [w643]
                            tunnel: w460 -> [w640]
                            tunnel: w463 -> [w641]
                            tunnel: w459 -> [w638]
                            tunnel: [w634] -> w450
                            tunnel: [w632] -> w449
                            tunnel: [w631] -> w447
                            tunnel: [w630] -> w446
                            tunnel: [w691] -> w462
                            tunnel: w450 -> [w689]
                            tunnel: w449 -> [w691]
                            tunnel: w447 -> [w686]
                            tunnel: w446 -> [w685]
                            tunnel: w462 -> [w715]
                            tunnel: [w714] -> w448
                            frame #0 {
                              # "Dir \nrow"
                              n228 = Increment(x=w468) -> (x+1=w477:dbl)
                              n229 = Increment(x=w476) -> (x+1=w479:dbl)
                              n230 = To Long Integer(number=w471) -> (32bit integer=w470:i32)
                              n231 = for {
                                N: w477 -> [_]
                                tunnel: w479 -> [w506]
                                shift-right: [w489] -> w482
                                shift-left: dbl[][] [] ("Intensity Graph") -> [w505]
                                shift-right: [w484] -> _
                                shift-left: FALSE -> [w492]
                                tunnel: w474 -> [w504]
                                tunnel: w475 -> [w503]
                                tunnel: w473 -> [w498]
                                tunnel: [w497] -> w478
                                tunnel: w477 -> [w495]
                                tunnel: w472 -> [w494]
                                tunnel: w470 -> [w493]
                                tunnel: w469 -> [w491]
                                tunnel: w468 -> [w486]
                                stop <- w502 stop-if-true
                                # "F - right,\n T - left"
                                n232 = flat-sequence {
                                tunnel: w506 -> [w516]
                                tunnel: w505 -> [w510]
                                tunnel: [w509] -> w489
                                tunnel: w492 -> [w511]
                                tunnel: w504 -> [w524]
                                tunnel: w503 -> [w523]
                                tunnel: [w518] -> w500
                                tunnel: [w519] -> w499
                                tunnel: w498 -> [w522]
                                tunnel: [w509] -> w496
                                tunnel: w495 -> [w521]
                                tunnel: w494 -> [w514]
                                tunnel: w493 -> [_]
                                tunnel: [w507] -> w484
                                tunnel: w500 -> [w595]
                                tunnel: w499 -> [w600]
                                tunnel: [w598] -> w497
                                tunnel: w496 -> [w597]
                                frame #0 {
                                # "Right/Left"
                                n233 = control-ref of="This VI"() -> (w520:refnum<vi>)
                                n234 = Increment(x=w516) -> (x+1=w517:dbl)
                                n235 = local read "Y_iter"() -> (w508:i32)
                                n236 = case shown="\"Phase\"" w522 {
                                tunnel: w516 -> [w568 w577]
                                tunnel: w524 -> [w576 w585]
                                tunnel: w523 -> [w575 w584]
                                tunnel: [w574 w583] -> w518
                                tunnel: [w573 w582] -> w519
                                tunnel: w521 -> [w571 w580]
                                tunnel: w508 -> [w570 w581]
                                tunnel: w520 -> [w572 w579]
                                tunnel: [w569 w578] -> w512
                                frame "Ampl", Default {
                                n237 = call "Scan read v_2 axis (SubVI).vi"("Y"=w570, "General VI"=w572, "error in (no error)"=w575, "Y_size"=w571, "X_size"=w568, "VISA Refnum in"=w576) -> ("error out"=w574:errorcluster, "value"=w569:dbl[], "VISA resource name out"=w573:refnum<visa-resource-name>)  [unwired: 3 in]
                                }
                                frame "Phase" {
                                n238 = call "Scan read phase v_2 axis (SubVI).vi"("Y"=w581, "General VI"=w579, "error in (no error)"=w584, "Y_size"=w580, "X_size"=w577, "VISA Refnum in"=w585) -> ("error out"=w583:errorcluster, "value"=w578:dbl[], "VISA Refnum out"=w582:refnum<visa-resource-name>)  [unwired: 2 in, 1 out]
                                }
                                }
                                n239 = Array Size(array=w512) -> (size(s)=w513:i32)
                                n240 = Greater?(x=w513, y=w517) -> (0:w515:bool)
                                n241 = case shown="True" w515 {
                                tunnel: w514 -> [w528 _]
                                tunnel: w513 -> [w533 w559]
                                tunnel: w512 -> [w532 w557]
                                tunnel: w511 -> [w526 w547]
                                tunnel: w510 -> [w529 w560]
                                tunnel: [w530 w561] -> w509
                                tunnel: w508 -> [w527 w548]
                                tunnel: [w525 w547] -> w507
                                frame False {
                                n242 = Reverse 1D Array(array=w532) -> (reversed array=w535:dbl[])
                                n243 = case shown="True" w528 {
                                tunnel: [w537 w546] -> w534
                                tunnel: w532 -> [w537 w544]
                                tunnel: w533 -> [_ w543]
                                tunnel: w535 -> [w538 w542]
                                tunnel: [w538 w540] -> w536
                                frame False {
                                }
                                frame True {
                                w539 = 0
                                n244 = Subtract(x=w543, y=w539) -> (x-y=w541:i32)
                                n245 = Delete From Array(array=w544, length=w539, index=0) -> (array with subset deleted=w546:dbl[])  [unwired: 1 out]
                                n246 = Delete From Array(array=w542, length=w539, index=w541) -> (array with subset deleted=w540:dbl[])  [unwired: 1 out]
                                }
                                }
                                n247 = Select(t=w536, s=w526, f=w534) -> (s? t:f=w531:dbl[])
                                n248 = Not(x=w526) -> (.not. x?=w525:bool)
                                n249 = Insert Into Array(array=w529, index (row)=w527, new element=w531) -> (w530:dbl[][])  [unwired: 1 in]
                                }
                                frame True {
                                # "if 2 row returns"
                                n250 = Divide(x=w559, y=2) -> (x/y=w556:dbl)
                                n251 = Array Subset(array=w557, index=w556, length=w556) -> (w555:dbl[])
                                n252 = Delete From Array(array=w557, length=w556, index=w556) -> (array with subset deleted=w554:dbl[])  [unwired: 1 out]
                                n253 = local read "Y_iter"() -> (w550:i32)
                                n254 = case shown="False" w547 {
                                tunnel: w555 -> [w564 w565]
                                tunnel: w554 -> [w562 w567]
                                tunnel: [w563 w565] -> w552
                                tunnel: [w562 w566] -> w553
                                frame False {
                                n255 = Reverse 1D Array(array=w564) -> (reversed array=w563:dbl[])
                                }
                                frame True {
                                n256 = Reverse 1D Array(array=w567) -> (reversed array=w566:dbl[])
                                }
                                }
                                n257 = Increment(x=w550) -> (x+1=w549:i32)
                                n258 = Build Array(w553, w552) -> (w551:dbl[][])
                                n259 = local write "Y_iter"(w549) -> ()
                                n260 = Insert Into Array(array=w560, index (row)=w548, new element=w551) -> (w561:dbl[][])  [unwired: 1 in]
                                }
                                }
                                "График интенсивности" <- w509
                                "Результат сканирования" <- w509
                                }
                                frame #1 {
                                w591 = 60 ("y")
                                # "Down"
                                n261 = call "Convert to Dynamic Data3"("2D Array"=w597) -> ("Dynamic Data Type"=w596:dynamicdata)  [unwired: 3 in]
                                n262 = local read "Y_iter"() -> (w590:i32)
                                n263 = local read "error in (no error)"() -> (w594:errorcluster)
                                n264 = call "Verify end axis (SubVI).vi"("error in"=w595, "VISA Refnum in"=w600) -> ("error out"=w598:errorcluster, "time, sec"=w593:i32, "progress, %"=→"Завершено, %":i32)  [unwired: 3 in, 1 out]
                                n265 = Quotient & Remainder(x=w593, y=w591) -> (x-y*floor(x/y)=→"Sec":i32, floor(x/y)=w592:i32)
                                n266 = Increment(x=w590) -> (x+1=→"Y_iter":i32)
                                n267 = Quotient & Remainder(x=w592, y=w591) -> (x-y*floor(x/y)=→"Min":i32, floor(x/y)=→"Hour":i32)
                                n268 = call "Backup1"("Signals"=w596, "error in (no error)"=w594) -> ()  [unwired: 15 in, 3 out]
                                }
                                }
                                n269 = local read "Y_iter"() -> (w487:i32)
                                n270 = Less Or Equal?(x=w486, y=w487) -> (x <= y?=w485:bool)
                                n271 = Equal?(x=0.0, y=w491) -> (x = y?=w488:bool)
                                n272 = local read "стоп"() -> (w501:bool)
                                n273 = Compound Arithmetic op=OR(w488, w497, w501, w485) -> (w502:bool)
                                "Dir_x" <- w492
                              }
                              n274 = local write "Диалоговое окно"("Сканирование... " ("Диалоговое окно")) -> ()
                            }
                            frame #1 {
                              n275 = local read "Частота излучения"() -> (w612:dbl)
                              n276 = local read "Толщина образца"() -> (w611:dbl)
                              n277 = local read "pos_no_sample"() -> (w610:dbl)
                              n278 = local read "начало Y, мм"() -> (w606:dbl)
                              n279 = local read "начало X, мм"() -> (w607:dbl)
                              n280 = local read "Шаг по X"() -> (w609:u32)
                              n281 = local read "Шаг по Y"() -> (w608:u32)
                              n282 = case shown="No Error" w605 {
                                tunnel: [w623 w626] -> w604
                                tunnel: [w624 w625] -> w603
                                frame No Error {
                                n283 = local read "конец X, мм"() -> (w623:dbl)
                                n284 = local read "конец Y, мм"() -> (w624:dbl)
                                }
                                frame Error {
                                n285 = local read "pos_xy"() -> (w627:cluster{"pos_x":dbl, "pos_y":dbl})
                                n286 = Unbundle(w627) -> ("pos_x"=w626:dbl, "pos_y"=w625:dbl)
                                }
                              }
                              n287 = local read "Режим\nсканирования"() -> (w602:enum32{"Ampl", "Phase"})
                              n288 = local read "конец X, мм"() -> (w613:dbl)
                              n289 = local read "конец Y, мм"() -> (w618:dbl)
                              n290 = case shown="\"Ampl\", Default" w602 {
                                tunnel: ["Ampl mode - " "Phase mode - "] -> w614
                                frame "Ampl", Default {
                                }
                                frame "Phase" {
                                }
                              }
                              n291 = local write "error out"(w605) -> ()
                              n292 = local read "P_ref"() -> (w601:dbl)
                              n293 = Select(t="Ошибка!" ("f"), s=w605, f="Сканирование завершено!" ("Диалоговое окно")) -> (s? t:f=→"Диалоговое окно":string)
                              n294 = Format Into String(format string="start pos(X:Y)=%f:%fmm, X=%fmm, step_X=%dum, Y=%fmm, step_Y=%dum, freq=%fGHz, d=%fmm, Xno_sample=%fmm, end position X:Y = %f:%f, P_reference=%f V. Comment: ", initial string=w614, w607, w606, w613, w609, w618, w608, w612, w611, w610, w604, w603, w601) -> (resulting string=w620:string)  [unwired: 1 in, 1 out]
                              n295 = Wait (ms)(milliseconds to wait=u32 1500) -> ()  [unwired: 1 out]
                            }
                            frame #2 {
                              n296 = Matrix Size(0:w644) -> (1:w636:i32, 2:w635:i32)
                              n297 = case shown="\"Phase\"" w641 {
                                tunnel: w644 -> [w647 w653]
                                tunnel: w643 -> [_ w659]
                                tunnel: w636 -> [_ w658]
                                tunnel: w640 -> [_ w657]
                                tunnel: w635 -> [_ w656]
                                tunnel: w638 -> [_ w655]
                                tunnel: "calc fi" -> [_ w654]
                                tunnel: [w646 w649] -> w632
                                tunnel: [FALSE TRUE] -> w630
                                frame "Ampl", Default {
                                n298 = call "Convert to Dynamic Data8"("2D Array"=w647) -> ("Dynamic Data Type"=w646:dynamicdata)  [unwired: 3 in]
                                }
                                frame "Phase" {
                                n299 = case shown="True" w654 {
                                tunnel: w653 -> [_ w667]
                                tunnel: w659 -> [_ w666]
                                tunnel: w658 -> [_ w665]
                                tunnel: w657 -> [_ w664]
                                tunnel: w656 -> [_ w663]
                                tunnel: [dbl[][] [] w662] -> w652
                                tunnel: w655 -> [_ w661]
                                frame False {
                                }
                                frame True {
                                n300 = for {
                                N: w665 -> [_]
                                tunnel: w667 -> [w673] mode=indexing
                                tunnel: w663 -> [w672]
                                tunnel: w666 -> [w671]
                                tunnel: w664 -> [w670]
                                tunnel: [w669] -> w662 mode=indexing
                                tunnel: w661 -> [w668]
                                n301 = for {
                                N: w672 -> [_]
                                tunnel: w673 -> [w681] mode=indexing
                                tunnel: w671 -> [w676]
                                tunnel: w670 -> [w680]
                                tunnel: [w679] -> w669 mode=indexing
                                tunnel: w668 -> [w677]
                                # "2pi*v*(Xs-Xns+d)"
                                n302 = Multiply(x=w681, y=w676) -> (x*y=w675:dbl)
                                n303 = Multiply(x=w676, y=w677) -> (x*y=w678:dbl)
                                n304 = Subtract(x=w675, y=w678) -> (x-y=w674:dbl)
                                n305 = Add(x=w674, y=w680) -> (x+y=w679:dbl)
                                }
                                }
                                }
                                }
                                n306 = call "Convert to Dynamic Data6"("2D Array"=w653) -> ("Dynamic Data Type"=w650:dynamicdata)  [unwired: 3 in]
                                n307 = call "Convert to Dynamic Data7"("2D Array"=w652) -> ("Dynamic Data Type"=w651:dynamicdata)  [unwired: 3 in]
                                n308 = Merge Signals(w650, w651) -> (w649:dynamicdata)
                                }
                              }
                              n309 = Concatenate Strings(w634, "Комментарий к файлу") -> (w642:string)
                              n310 = call "Backup"("Signals"=w632, "error in (no error)"="error in (no error)", "Comment"=w642) -> ("error out"=w631:errorcluster)  [unwired: 14 in, 2 out]
                            }
                            frame #3 {
                              w690 = FALSE ("start scaning")
                              n311 = Select(t="После сохранения незабудьте измерить\nОПОРНЫЙ СИГНАЛ С ДЕТЕКТОРА!", s=w685, f="") -> (s? t:f=w683:string)
                              n312 = local write "start scaning"(w690) -> ()
                              n313 = Concatenate Strings("Выберите имя файла с результатами и путь\nи нажмите Сохранить или нажмите Не сохранять.\n" ("Диалоговое окно"), w683) -> (w687:string)
                              n314 = while {
                                tunnel: [w703] -> w692
                                tunnel: w691 -> [w700]
                                tunnel: w686 -> [w699]
                                tunnel: w689 -> [w698]
                                tunnel: w687 -> [w695]
                                stop <- w702 stop-if-true
                                n315 = local read "Комментарий к файлу"() -> (w696:string)
                                n316 = Concatenate Strings(w698, w696) -> (w697:string)
                                n317 = case shown="True" "сохр" {
                                tunnel: "Имя файла с результатами" -> [_ w713]
                                tunnel: w700 -> [_ w708]
                                tunnel: ["отмена" w712] -> w702
                                tunnel: [FALSE w712] -> w703
                                tunnel: w697 -> [_ w709]
                                tunnel: w699 -> [w705 w711]
                                frame False {
                                n318 = local write "error out"(w705) -> ()
                                }
                                frame True {
                                n319 = call "Save"("Signals"=w708, "error in (no error)"=w711, "Filename"=w713, "Comment"=w709) -> ("Saving Data"=w712:bool, "error out"=→"error out":errorcluster)  [unwired: 13 in, 1 out]
                                }
                                }
                                n320 = local write "Диалоговое окно"(w695) -> ()
                              }
                              n321 = case shown="True" w692 {
                                frame False {
                                }
                                frame True {
                                n322 = local write "Диалоговое окно"("Результаты сохранены в файл!" ("Диалоговое окно")) -> ()
                                n323 = Wait (ms)(milliseconds to wait=u32 1500) -> ()  [unwired: 1 out]
                                }
                              }
                              n324 = local write "стоп"(w690) -> ()
                            }
                            frame #4 {
                              w716 = FALSE ("отмена")
                              n325 = local write "отмена"(w716) -> ()
                              n326 = local write "сохр"(w716) -> ()
                              n327 = call "Convert from Dynamic Data"("Dynamic Data Type"=w715) -> ("Array"=w714:dbl[][])  [unwired: 3 in]
                            }
                          }
                        }
                        frame Error {
                          w717 = FALSE ("стоп")
                          n328 = local write "start scaning"(w717) -> ()
                          n329 = local write "стоп"(w717) -> ()
                        }
                      }
                    }
                  }
                }
              }
              n330 = local read "start scaning"() -> (w40:bool)
              n331 = local read "стоп"() -> (w39:bool)
              n332 = And(x=w40, y=w39) -> (x .and. y?=w38:bool)
            }
          }
          frame #1 {
            n333 = local read "error in (no error)"() -> (w719:errorcluster)
            n334 = local write "Диалоговое окно"("Остановлено!" ("Диалоговое окно")) -> ()
            n335 = local write "стоп"(FALSE ("стоп")) -> ()
            n336 = Wait (ms)(milliseconds to wait=u32 1000) -> ()  [unwired: 1 out]
          }
          frame #2 {
            w726 = FALSE ("сохр")
            n337 = while {
              tunnel: w725 -> [w729]
              tunnel: [w728] -> w724
              stop <- w736 stop-if-true
              n338 = local read "сохр"() -> (w732:bool)
              n339 = local read "Имя файла с результатами"() -> (w733:path)
              n340 = local read "Комментарий к файлу"() -> (w730:string)
              n341 = case shown="True" w732 {
                tunnel: w733 -> [_ w744]
                tunnel: w730 -> [_ w742]
                tunnel: [FALSE w743] -> w731
                tunnel: w729 -> [w737 w740]
                tunnel: [w737 w739] -> w728
                frame False {
                }
                frame True {
                  n342 = local read "Результат сканирования"() -> (w741:T1)
                  n343 = call "Convert to Dynamic Data4"("2D Array"=w741) -> ("Dynamic Data Type"=w745:dynamicdata)  [unwired: 3 in]
                  n344 = call "Save stop"("Signals"=w745, "error in (no error)"=w740, "Filename"=w744, "Comment"=w742) -> ("Saving Data"=w743:bool, "error out"=w739:errorcluster)  [unwired: 13 in, 1 out]
                }
              }
              n345 = local read "отмена"() -> (w735:bool)
              n346 = local write "Диалоговое окно"("Сохранить результаты?" ("Диалоговое окно")) -> ()
              n347 = Or(x=w731, y=w735) -> (x .or. y?=w736:bool)
            }
            n348 = local write "сохр"(w726) -> ()
            n349 = local write "сохр"(w726) -> ()
          }
          frame #3 {
            w748 = FALSE
            n350 = local write "отмена"(w748) -> ()
            n351 = Matrix Size(0:w750) -> (1:w752:i32)  [unwired: 1 out]
            n352 = local write "Завершено, %"(0.0 ("Завершено, %")) -> ()
            n353 = local write "error out"(w747) -> ()
            n354 = local write "сохр"(w748) -> ()
            n355 = Delete From Array(array=w750, length=w752, index (row)=0 ("disabled index (col)")) -> (array with subset deleted=w749:dbl[][])  [unwired: 1 in, 1 out]
            n356 = local write "Результат сканирования"(w749) -> ()
            n357 = local write "График интенсивности"(w749) -> ()
          }
        }
      }
    }
    frame Error {
    }
  }
  n358 = local read "Dir_x"() -> (w2:bool)
  n359 = node-c288(i64 1 ("Period"), 2 ("Priority")) -> (w8:T2)  [unwired: 2 in]
  n360 = Not(x=w2) -> (.not. x?=w1:bool)
  n361 = timed-loop {
    timing: w8 -> [_]
    timing-out: [_] -> w7
    shift-right: [w758] -> _
    shift-left: w3 -> [w757]
    shift-right: [w756] -> _
    shift-left: w3 -> [w755]
    shift-right: [w754] -> _
    shift-left: w1 -> [w753]
    stop <- _ stop-if-true
    n362 = node-c288() -> (w759:errorcluster)  [unwired: 1 in]
    n363 = local read "start scaning"() -> (w760:bool)
    n364 = global write "GlobalStop.vi" "Гл.Стоп"("стоп") -> ()
    n365 = case shown="True" w760 {
      tunnel: [w765 w789] -> w758
      tunnel: w757 -> [w763 w786]
      tunnel: [w765 w779] -> w756
      tunnel: w755 -> [w764 w782]
      tunnel: [w762 w776] -> w754
      tunnel: w753 -> [w762 w777]
      frame False {
        w765 = 0 ("Y_iter")
        n366 = local write "X_iter"(w764) -> ()
        n367 = local write "Y_iter"(w763) -> ()
      }
      frame True {
        w788 = 1000.0 ("y")
        n368 = local read "Шаг по Y"() -> (w781:u32)
        n369 = local read "Шаг по X"() -> (w796:u32)
        n370 = local read "Y_iter"() -> (w787:i32)
        n371 = local read "Dir_x"() -> (w792:bool)
        n372 = local read "конец X, мм"() -> (w769:dbl)
        n373 = local read "начало X, мм"() -> (w768:dbl)
        n374 = Not(x=w792) -> (.not. x?=w770:bool)
        n375 = Not Equal?(x=w777, y=w770) -> (x != y?=w778:bool)
        n376 = local read "pos_xy"() -> (w780:cluster{"pos_x":dbl, "pos_y":dbl})
        n377 = Divide(x=w796, y=w788) -> (x/y=w771:dbl)
        n378 = Divide(x=w781, y=w788) -> (x/y=w794:dbl)
        n379 = Greater?(x="X_iter", y=w782) -> (0:w783:bool)
        n380 = Greater?(x=w787, y=w786) -> (0:w785:bool)
        n381 = Unbundle(w780) -> ("pos_x"=w791:dbl, "pos_y"=w795:dbl)
        n382 = case shown="True" w785 {
          tunnel: w795 -> [w839 w846]
          tunnel: w794 -> [_ w845]
          tunnel: [w839 w840] -> w793
          tunnel: w787 -> [_ w844]
          tunnel: [w838 w844] -> w789
          tunnel: w786 -> [w838 _]
          frame False {
          }
          frame True {
            n383 = Add(x=w846, y=w845) -> (x+y=w842:dbl)
            n384 = local read "конец Y, мм"() -> (w841:dbl)
            n385 = Less Or Equal?(x=w842, y=w841) -> (x <= y?=w843:bool)
            n386 = Select(t=w842, s=w843, f=w841) -> (s? t:f=w840:dbl)
          }
        }
        n387 = case shown="True" w783 {
          tunnel: w770 -> [w828 w831]
          tunnel: [w830 w836] -> w775
          tunnel: w791 -> [w830 w834]
          tunnel: w771 -> [_ w833]
          tunnel: "X_iter" -> [_ w832]
          tunnel: [w829 w832] -> w773
          tunnel: w782 -> [w829 _]
          tunnel: [w828 w831] -> w776
          frame False {
          }
          frame True {
            n388 = Add(x=w833, y=w834) -> (x+y=w837:dbl)
            n389 = Subtract(x=w834, y=w833) -> (x-y=w835:dbl)
            n390 = Select(t=w837, s=w831, f=w835) -> (s? t:f=w836:dbl)
          }
        }
        n391 = case shown="False" w778 {
          tunnel: w770 -> [w801 w810]
          tunnel: w775 -> [w800 _]
          tunnel: [w799 w811] -> w774
          tunnel: w773 -> [w806 _]
          tunnel: [w806 0 ("X_iter")] -> w772
          tunnel: w769 -> [w804 w808]
          tunnel: w768 -> [w802 w807]
          frame False {
            n392 = Greater?(x=w800, y=w804) -> (0:w805:bool)
            n393 = Select(t=w804, s=w805, f=w800) -> (s? t:f=w797:dbl)
            n394 = Greater?(x=w802, y=w800) -> (0:w803:bool)
            n395 = Select(t=w802, s=w803, f=w800) -> (s? t:f=w798:dbl)
            n396 = Select(t=w797, s=w801, f=w798) -> (s? t:f=w799:dbl)
          }
          frame True {
            n397 = Select(t=w807, s=w810, f=w808) -> (s? t:f=w811:dbl)
          }
        }
        n398 = local read "X_iter"() -> (w767:i32)
        n399 = case shown="False" w776 {
          tunnel: w774 -> [w816 w827]
          tunnel: w769 -> [_ w826]
          tunnel: w772 -> [w817 w825]
          tunnel: [w813 w820] -> w779
          tunnel: w768 -> [w815 _]
          tunnel: w767 -> [w814 w821]
          tunnel: [w813 w820] -> w766
          frame False {
            n400 = Less Or Equal?(x=w816, y=w815) -> (x <= y?=w819:bool)
            n401 = Select(t=0, s=w819, f=w817) -> (s? t:f=w812:i32)
            n402 = Select(t=w812, s=w819, f=w814) -> (s? t:f=w813:i32)
          }
          frame True {
            n403 = Greater Or Equal?(x=w827, y=w826) -> (x >= y?=w823:bool)
            n404 = Select(t=0, s=w823, f=w825) -> (s? t:f=w822:i32)
            n405 = Select(t=w822, s=w823, f=w821) -> (s? t:f=w820:i32)
          }
        }
        n406 = Bundle(cluster=w780, "pos_x"=w774, "pos_y"=w793) -> (w790:cluster{"pos_x":dbl, "pos_y":dbl})
        n407 = local write "pos_xy"(w790) -> ()
        n408 = local write "X_iter"(w766) -> ()
      }
    }
    n409 = node-c288(w759) -> ()  [unwired: 1 out]
  }
  n410 = node-c288(w7) -> ()  [unwired: 1 out]
